vi "Msg.vi"(7 "Queue Actor in":refnum<class "Queue Actor.lvclass">, 11 "Teardown Msg in":refnum<class "Teardown Msg.lvclass">) -> (5 "Queue Actor out":refnum<class "Queue Actor.lvclass">)   [LabVIEW 2021, in "Teardown.lvlib" / "Teardown Msg.lvclass"]
uses:
  Teardown Msg.lvclass
  Queue Actor/Queue Actor.lvclass
  Teardown/Teardown.lvclass
  8b074ebc-55b2-44bc-a317-0de79f881938.vi
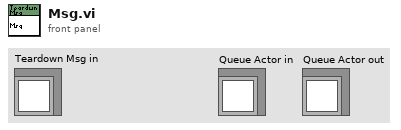
[diagram p1: front panel]
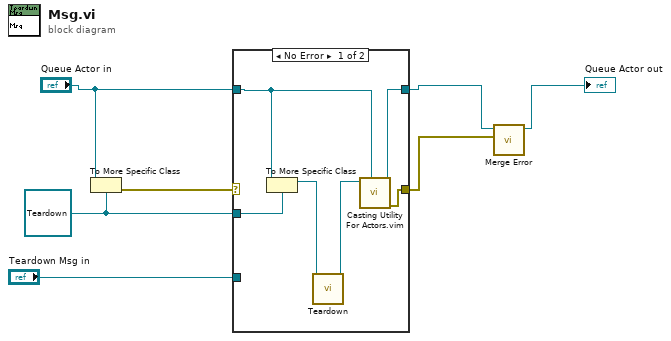
[diagram p0: block diagram]
diagram:
  w4 = refnum<class "Teardown.lvclass"> refnum ("Destroy.lvlib:Destroy.lvclass")
  n1 = To More Specific Class(target class=w4, reference="Queue Actor in") -> (error out=w7:errorcluster)  [unwired: 1 in, 1 out]
  n2 = case shown="No Error" w7 {
    selector: w7 -> [_ w14]
    tunnel: [w12 w15] -> w3
    tunnel: "Queue Actor in" -> [w11 w15]
    tunnel: w4 -> [w13 _]
    tunnel: "Teardown Msg in" -> [_ _]
    tunnel: [w8 w14] -> w1
    frame No Error {
      n3 = To More Specific Class(target class=w13, reference=w11) -> (specific class reference=w10:refnum<class "Teardown.lvclass">)  [unwired: 1 in, 1 out]
      n4 = call-dynamic "Teardown.vi"("Teardown in"=w10) -> ("Teardown out"=w9:refnum<class "Teardown.lvclass">)  [unwired: 10 in]
      n5 = call "Casting Utility For Actors.vim"("type"=w11, "Actor in"=w9) -> ("error out"=w8:errorcluster, "Actor out"=w12:refnum<class "Queue Actor.lvclass">)  [unwired: 8 in]
    }
    frame Error {
    }
  }
  n6 = call-dynamic "Merge Error.vi"("Error"=w1, "Set Error in"=w3) -> ("Set Error out"=→"Queue Actor out":refnum<class "Queue Actor.lvclass">)  [unwired: 9 in]
